vi "ceg_number_to_string_format.vi"(0 "Counter":i32, 3 "erro in":errorcluster) -> (7 "out":string, 10 "error out":errorcluster)   [LabVIEW 2013, in "Spannungseinbruch.lvclass"]
uses:
  Tests/Spannungseinbruch/Spannungseinbruch.lvclass
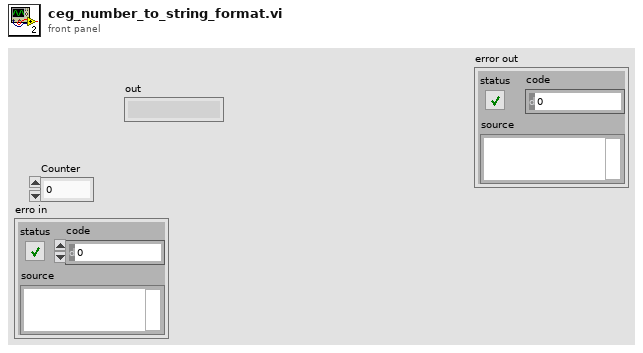
[diagram p1: front panel]
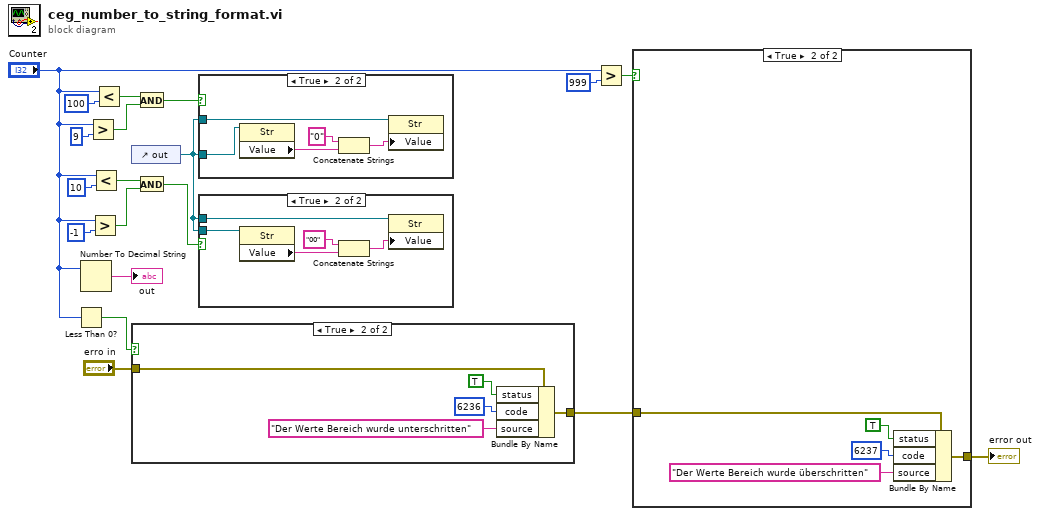
[diagram p0: block diagram]
diagram:
  n1 = Less Than 0?(x="Counter") -> (x < 0?=w3:bool)
  n2 = Number To Decimal String(number="Counter") -> (decimal integer string=→"out":string)  [unwired: 1 in]
  n3 = Greater?(x="Counter", y=9) -> (0:w15:bool)
  n4 = Greater?(x="Counter", y=-1) -> (0:w16:bool)
  n5 = Less?(x="Counter", y=10) -> (x < y?=w18:bool)
  n6 = Less?(x="Counter", y=100) -> (x < y?=w13:bool)
  n7 = control-ref of="out"() -> (w6:refnum<vi>)
  n8 = case shown="True" w3 {
    tunnel: "erro in" -> [w20 w22]
    tunnel: [w20 w21] -> w1
    frame False {
    }
    frame True {
      n9 = Bundle By Name(cluster=w22, "status"=TRUE, "code"=6236, "source"="Der Werte Bereich wurde unterschritten") -> (w21:errorcluster)
    }
  }
  n10 = And(x=w13, y=w15) -> (x .and. y?=w8:bool)
  n11 = And(x=w18, y=w16) -> (x .and. y?=w9:bool)
  n12 = case shown="True" w8 {
    tunnel: w6 -> [_ w27]
    tunnel: w6 -> [_ w26]
    frame False {
    }
    frame True {
      n13 = property class="Str"(reference=w26) -> ("Value"=w28:string)  [unwired: 1 in, 2 out]
      n14 = Concatenate Strings("0" ("string"), w28) -> (w29:string)
      n15 = property class="Str"(reference=w27, "Value"=w29) -> ()  [unwired: 1 in, 2 out]
    }
  }
  n16 = case shown="True" w9 {
    tunnel: w6 -> [_ w32]
    tunnel: w6 -> [_ w31]
    frame False {
    }
    frame True {
      n17 = property class="Str"(reference=w31) -> ("Value"=w33:string)  [unwired: 1 in, 2 out]
      n18 = Concatenate Strings("00" ("string"), w33) -> (w35:string)
      n19 = property class="Str"(reference=w32, "Value"=w35) -> ()  [unwired: 1 in, 2 out]
    }
  }
  n20 = Greater?(x="Counter", y=999) -> (0:w7:bool)
  n21 = case shown="True" w7 {
    tunnel: w1 -> [w36 w41]
    tunnel: [w36 w37] -> w5
    frame False {
      # "fehler"
    }
    frame True {
      n22 = Bundle By Name(cluster=w41, "status"=TRUE, "code"=6237, "source"="Der Werte Bereich wurde überschritten") -> (w37:errorcluster)
    }
  }
  "error out" <- w5
